vi "LibCam_GetImage.vi"(8 "error in (no error)":errorcluster) -> (0 "error out":errorcluster, 1 "height":i32, 2 "width":i32, 3 "return type":i32)   [LabVIEW 2014, in "QwaveSys Raspberry Pi Library.lvlib"]
uses:
  QwaveSys Raspberry Pi Library.lvlib
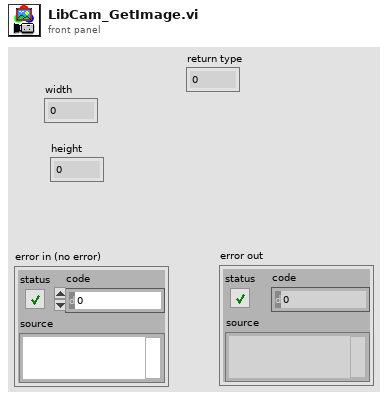
[diagram p1: front panel]
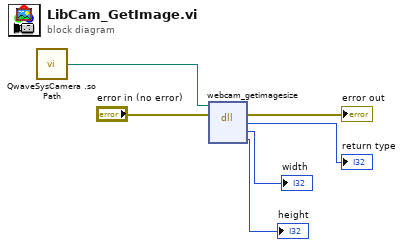
[diagram p0: block diagram]
diagram:
  n1 = call "QwaveSysCamera .so Path.vi"() -> ("QwaveSys .so Path"=w6:path)  [unwired: 5 in]
  n2 = dll-call lib="libcamera.so" fn="webcam_getimagesize"(path in=w6, error in="error in (no error)") -> (error out=→"error out":errorcluster, "return type"=→"return type":i32, "w"=→"width":i32, "h"=→"height":i32)  [unwired: 3 in, 1 out]
